vi "Read Status Byte.vi"(8 "error in (no error)":errorcluster, 11 "SR3XXX HVPS in":refnum<class "SR3XXX HVPS.lvclass">) -> (0 "error out":errorcluster, 2 "Byte":bool[](array[boolean]), 3 "SR3XXX HVPS out":refnum<class "SR3XXX HVPS.lvclass">)   [LabVIEW 2014, in "SR3XXX HVPS.lvclass"]
doc: "The *STB? common command query reads the value of the serial poll status byte. If the optional parameter i is present, the value of bit i is returned. Reading this register will clear bits 1, 2, and 3; the remaining bits are either real-time monitors of underlying conditions (such as bit 7: HVON), or summary bits (such as\nbit 5: ESB).\n\nBit (Name) Usage\n=============\n0 (stable) Indicates VSET or ILIM value is stable. The value depends on whether the PS300 is in constant current or constant voltage mode.\n1 (vtrip) Indicates a voltage trip has occurred\n2 (itrip) Indicates a current trip has occurred\n3 (ilim) Indicates a current limit condition has occurred\n4 (MAV) Indicates GPIB output queue is non-empty\n5 (ESB) Indicates an unmasked bit in the standard status byte has been set\n6 (RQS/MSS) SRQ bit\n7 (hvon) Indicates high voltage is on\n\nThe PS300 will make a service request (SRQ) whenever one of these bits is set and the corresponding bit in the serial poll enable register is set. Note that any status condition will produce only one SRQ even if it is never cleared. The vtrip, itrip and ilim bits are latched bits. They are set on the occurrence of the appropriate event and stay set until either the status byte is read or the *CLS command is sent. This allows one to detect if a trip condition has ever occurred. All the other bits indicate the current states of their respective functions."
uses:
  SR3XXX HVPS.lvclass
  reusable/Session APIs/Serial/Typedefs/Session Handle.ctl
  reusable/Session APIs/Serial/Serial Session.lvclass
  Base/Session HVPS.lvclass/Session HVPS.ctl
  Base/Read hSession.vi
  reusable/Session APIs/Serial/Public/Asynchronous Write.vi
  reusable/Session APIs/Serial/Public/Asynchronous Read.vi
  <userlib>/_Session Fwk/Session - Root.lvclass
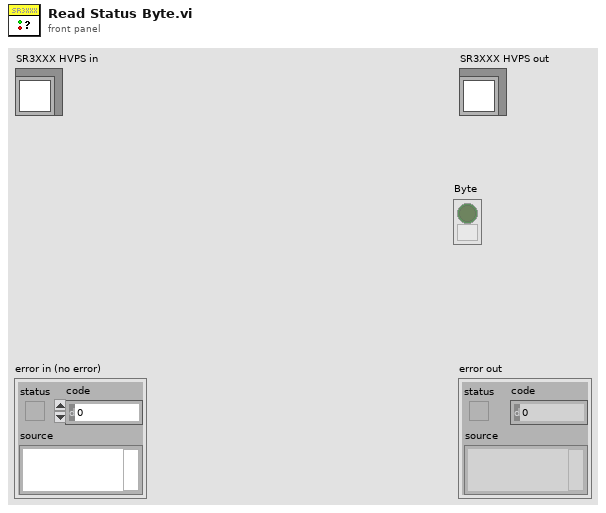
[diagram p1: front panel]
types:
  T1 = typedef "Serial Session.lvclass/Session Handle.ctl" = refnum<data-value>
  T2 = typedef "Session - Root.lvclass/Session Handle.ctl" = refnum<data-value>
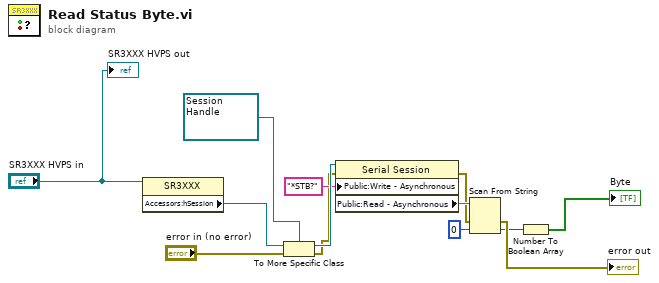
[diagram p0: block diagram]
diagram:
  n1 = property class="SR3XXX"(reference="SR3XXX HVPS in") -> ("Accessors:hSession"=w12:T2)  [unwired: 1 in, 2 out]
  n2 = To More Specific Class(target class=T1 refnum ("Session Handle"), reference=w12, error in="error in (no error)") -> (specific class reference=w10:T1, error out=w6:errorcluster)
  n3 = property class="Serial Session"(reference=w10, error in=w6, "Public:Write - Asynchronous"="*STB?" ("Cmd")) -> (error out=w5:errorcluster, "Public:Read - Asynchronous"=w8:string)  [unwired: 1 out]
  n4 = Scan From String(input string=w8, error in=w5, default 1=u8 0 ("default value 1")) -> (error out=→"error out":errorcluster, output 1=w2:u8)  [unwired: 2 in, 2 out]
  n5 = Number To Boolean Array(number=w2) -> (Boolean array=→"Byte":bool[])
  "SR3XXX HVPS out" <- "SR3XXX HVPS in"
